vi "GetCounterTime.vi"(10 "CtrNum":u8, 11 "error in":errorcluster caption="错误输入") -> (2 "CounterTime":dbl, 3 "error out":errorcluster caption="错误输出")   [LabVIEW 2016]
uses:
  PLC-Lab/lib/gusb.dll
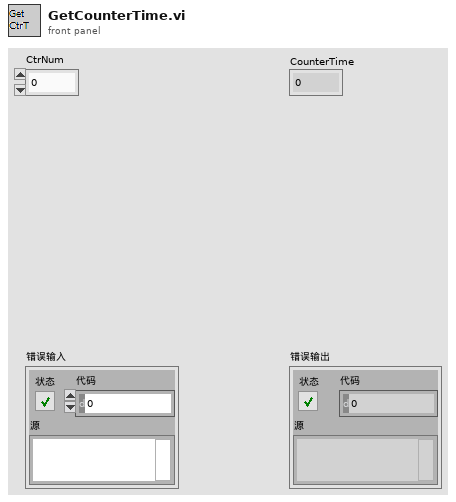
[diagram p1: front panel]
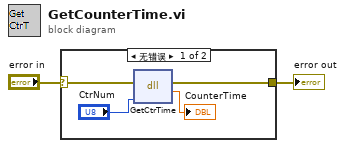
[diagram p0: block diagram]
diagram:
  n1 = case shown="无错误" "error in" {
    selector: "error in" -> [w6 w7]
    tunnel: [w5 w7] -> w1
    frame No Error {
      n2 = dll-call lib="E:/Camproject/2018/2018.1Labview/PLC-Lab/lib/gusb.dll" fn="GetCtrTime"(error in=w6, "CtrNum"="CtrNum") -> (error out=w5:errorcluster, "CounterTime"=→"CounterTime":dbl)  [unwired: 3 in, 1 out]
    }
    frame Error {
    }
  }
  "error out" <- w1
